vi "Destroy DO DAQmx Refs.vi"(8 "error in (no error)":errorcluster, 10 "DO":T1) -> (0 "error out":errorcluster, 2 "DO out":T1)   [LabVIEW 2017, in "DAQ.lvclass"]
doc: "Developed by Kevin Thompson\nkevin@thompsonengineering.net\n\nCopyright 2018-2020\nThompson Engineering, LLC"
uses:
  DAQ.lvclass
  DataTypes/TD DO Channel--cluster.ctl
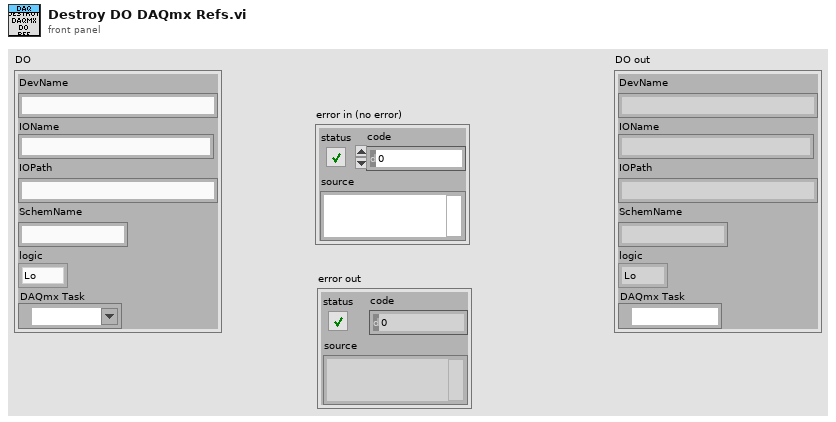
[diagram p1: front panel]
types:
  T1 = typedef "DAQ.lvclass/TD DO Channel--cluster.ctl" = cluster{"DevName":string, "IOName":string, "IOPath":string, "SchemName":string, "logic":enum16{"Lo", "Hi"}, "DAQmx Task":refnum<k21>}
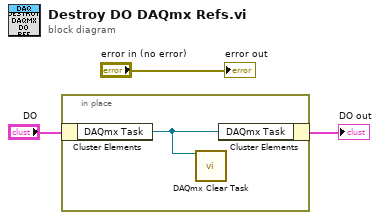
[diagram p0: block diagram]
diagram:
  n1 = in-place {
    n2 = in-place-cluster #1("DO") -> ("DAQmx Task"=w4:refnum<k21>)
    n3 = call <vilib>:"DAQmx Clear Task.vi"("task in"=w4) -> ()  [unwired: 14 in, 1 out]
    n4 = in-place-cluster #1("DAQmx Task"=w4) -> (→"DO out":T1)
  }
  "error out" <- "error in (no error)"
